vi "Serial Main.vi"(8 "error in (no error)":errorcluster, 9 "Write":bool, 10 "Command":string="*IDN?", 11 "Alias":string="FTDI") -> (0 "error out":errorcluster={"status"=TRUE, "code"=-1073807346, "source"="VISA Clear in Wrappers.lvlib:Serial.vi->Wrappers.lvlib:Serial Main.vi"}, 3 "Output":string)   [LabVIEW 2021, in "Wrappers.lvlib"]
uses:
  Wrappers.lvlib
  Controls/Serial States.ctl
panel:
  in  "stop":bool
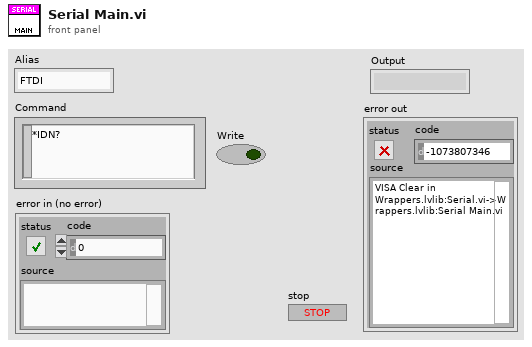
[diagram p1: front panel]
types:
  T1 = typedef "Wrappers.lvlib/Serial States.ctl" = enum16{"Init", "Read", "Write", "Close"}
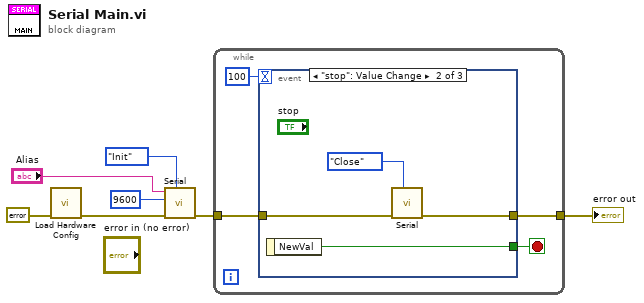
[diagram p0: block diagram]
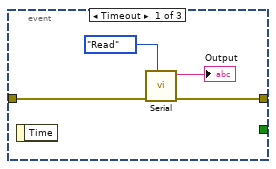
[diagram p2: hidden frame]
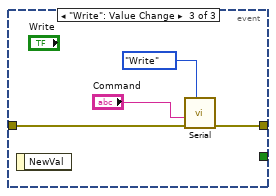
[diagram p3: hidden frame]
diagram:
  n1 = call "Load Hardware Config.vi"("error in"=errorcluster {"status"=FALSE, "code"=0, "source"=""}) -> ("error out"=w3:errorcluster)  [unwired: 10 in]
  n2 = call "Serial.vi"("States"=Serial_States."Init", "error in"=w3, "baud rate"=u32 9600, "Alias"="Alias") -> ("error out"=w1:errorcluster)  [unwired: 6 in, 1 out]
  n3 = while {
    tunnel: w1 -> [w10]
    tunnel: [w9] -> w6
    stop <- w11 stop-if-true
    n4 = event shown="[1] \"stop\": Value Change" {
      selector: _ -> [_ _ _]
      dyn-events: _ -> [_ _ _]
      timeout: 100 -> [_ _ _]
      tunnel: [_ w19 _] -> w11
      tunnel: [w14 w17 w22] -> w9
      tunnel: w10 -> [w15 w18 w23]
      event Timeout {
        n5 = event-data() -> ()  [unwired: 1 in, 1 out]
        n6 = call "Serial.vi"("States"=Serial_States."Read", "error in"=w15) -> ("error out"=w14:errorcluster, "Output"=→"Output":string)  [unwired: 8 in]
      }
      event "stop": Value Change {
        n7 = event-data() -> ("NewVal"=w19:bool)  [unwired: 1 in]
        n8 = call "Serial.vi"("States"=Serial_States."Close", "error in"=w18) -> ("error out"=w17:errorcluster)  [unwired: 8 in, 1 out]
      }
      event "Write": Value Change {
        n9 = event-data() -> ()  [unwired: 1 in, 1 out]
        n10 = call "Serial.vi"("States"=Serial_States."Write", "error in"=w23, "Command"="Command") -> ("error out"=w22:errorcluster)  [unwired: 7 in, 1 out]
      }
    }
  }
  "error out" <- w6
